vi "Destroy.vi"(8 "error in (no error)":errorcluster, 11 "(WavBuf) in":refnum<class "(WavBuf).lvclass">) -> (0 "error out":errorcluster, 3 "(WavBuf)":refnum<class "(WavBuf).lvclass">)   [LabVIEW 2016, in "(WavBuf).lvclass"]
uses:
  (WavBuf).lvclass
  (WavBuf).lvclass/(WavBuf).ctl
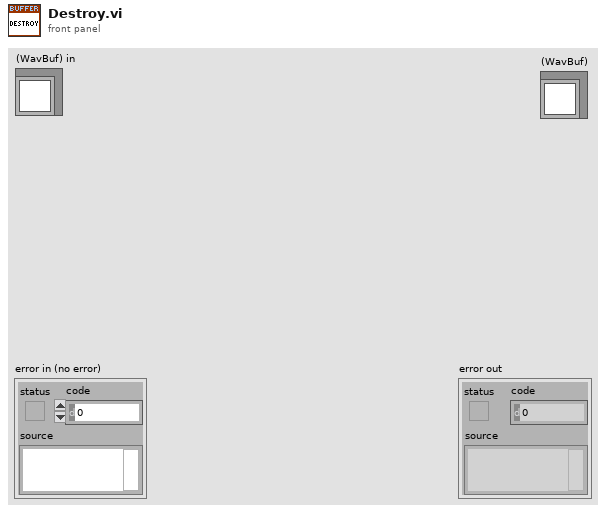
[diagram p1: front panel]
types:
  T1 = typedef "Ref_DVR_Buffer.ctl" = refnum<data-value>
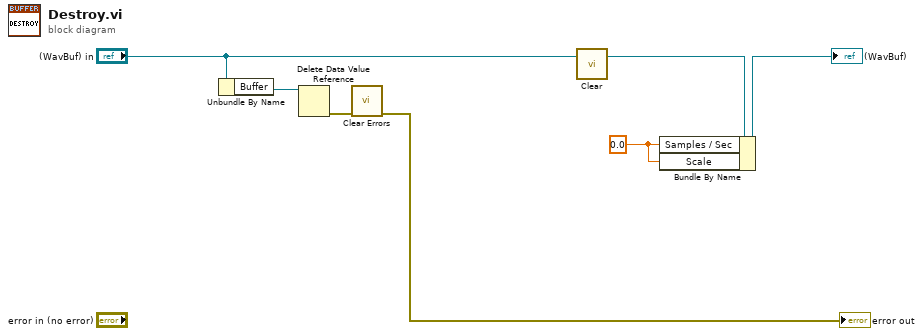
[diagram p0: block diagram]
diagram:
  w1 = 0.0 ("Samples / Sec")
  n1 = Unbundle By Name("(WavBuf) in") -> ("Buffer"=w5:T1)
  n2 = Delete Data Value Reference(data value reference=w5) -> (error out=w4:errorcluster)  [unwired: 1 in, 1 out]
  n3 = call <vilib>:"Clear Errors.vi"("error in (no error)"=w4) -> ("error out"=→"error out":errorcluster)  [unwired: 5 in, 1 out]
  n4 = call-dynamic "Clear.vi"("(WavBuf)"="(WavBuf) in") -> ("(WavBuf) Out"=w3:refnum<class "(WavBuf).lvclass">)  [unwired: 2 in]
  n5 = Bundle By Name(cluster=w3, "Samples / Sec"=w1, "Scale"=w1) -> (→"(WavBuf)":refnum<class "(WavBuf).lvclass">)
